vi "DTL_Query.vi"(0 "System no.":i32=1 min=1 max=4 step=1, 2 "DDL table  to query":i32[](array[numeric]), 3 "All tables?":bool, 5 "error in":errorcluster) -> (14 "Table length":dbl[](array[numeric]) format="%.6f", 19 "error out":errorcluster)   [LabVIEW 2020]
doc: "Returns DDL table length."
panel:
  # "Returns DDL table length."
  # "Query"
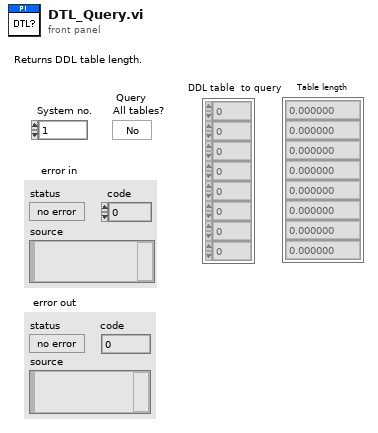
[diagram p1: front panel]
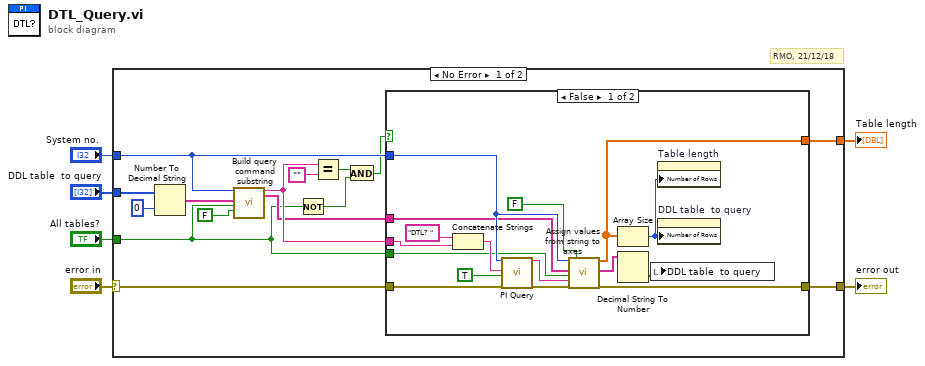
[diagram p0: block diagram]
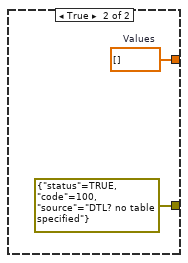
[diagram p2: hidden frame]
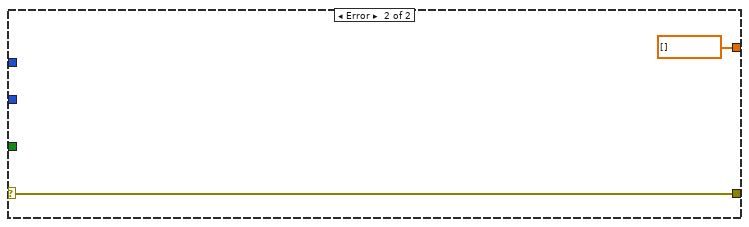
[diagram p3: hidden frame]
diagram:
  # "RMO, 21/12/18"
  n1 = case shown="No Error" "error in" {
    selector: "error in" -> [w7 w40]
    tunnel: [w15 dbl[] [] ("Values")] -> w6
    tunnel: "DDL table  to query" -> [w11 _]
    tunnel: [w9 w40] -> w4
    tunnel: "System no." -> [w19 _]
    tunnel: "All tables?" -> [w13 _]
    frame No Error {
      n2 = Number To Decimal String(number=w11, width (-)=i16 0) -> (decimal integer string=w10:string[])
      n3 = call "Build query command substring.vi"("System no."=w19, "Axes to query in"=w10, "Query\nAll axes?"=w13, "For all axes: use\nAxis identifier?"=FALSE ("For all axes: use\nAxis identifier?")) -> ("Command substring"=w20:string, "Axes to query out"=w18:string[])  [unwired: 2 in, 12 out]
      n4 = Not(x=w13) -> (.not. x?=w17:bool)
      n5 = Equal?(x=w20, y="" ("x")) -> (x = y?=w16:bool)
      n6 = And(x=w16, y=w17) -> (x .and. y?=w8:bool)
      n7 = case shown="False" w8 {
        tunnel: w20 -> [w34 _]
        tunnel: w19 -> [w33 _]
        tunnel: w18 -> [w32 _]
        tunnel: [w31 w38] -> w15
        tunnel: w13 -> [w29 _]
        tunnel: w7 -> [w25 _]
        tunnel: [w24 errorcluster {"status"=TRUE, "code"=100, "source"="DTL? no table specified"} ("error out")] -> w9
        frame False {
          n8 = Concatenate Strings("DTL? ", w34) -> (w35:string)
          n9 = call "PI Query.vi"("System no."=w33, "String to send"=w35, "Attach termination char.?"=TRUE ("Attach Linefeed?"), "error in"=w25) -> ("String read"=w22:string, "error out"=w23:errorcluster)  [unwired: 3 in, 11 out]
          n10 = call "Assign values from string to axes.vi"("System no."=w33, "Queried axes"=w32, "All axes queried?"=w29, "Input String"=w22, "error in"=w23, "Axes related?"=FALSE) -> ("Values"=w31:dbl[], "Queried axes out"=w27:string[], "error out"=w24:errorcluster)  [unwired: 3 in, 8 out]
          n11 = Array Size(array=w31) -> (size(s)=w28:i32)
          n12 = Decimal String To Number(string=w27) -> (number=w26:i32[])  [unwired: 3 out]
          n13 = local write "DDL table  to query"(w26) -> ()
          n14 = property on="Table length" class="Arr (strict)"("Number of Rows"=w28) -> ()  [unwired: 2 in, 2 out]
          n15 = property on="DDL table  to query" class="Arr (strict)"("Number of Rows"=w28) -> ()  [unwired: 2 in, 2 out]
        }
        frame True {
          w38 = dbl[] []  # Values
        }
      }
    }
    frame Error {
    }
  }
  "error out" <- w4
  "Table length" <- w6
